vi "Channel 0 Timer And Data Read (SubVI).vi"(5 "BoardHandle in":T1, 7 "Channel # in":i32, 11 "error in (no error)":errorcluster) -> (1 "Actual Voltage Level (V)":dbl format="%#_13g", 2 "Power Supply Trip":bool, 3 "Actual Current Limit (nA)":dbl format="%#_13g", 10 "Array":dbl[](array[numeric]), 14 "BoardHandle out 2":T1, 15 "error out":errorcluster)   [LabVIEW 2020]
uses:
  SUB VI Dark Current Test Files 2018 For Drop Box/Program Files (x86)/National Instruments/LabVIEW 2020/instr.lib/CAEN PSM/CAEN PSM.lvlib
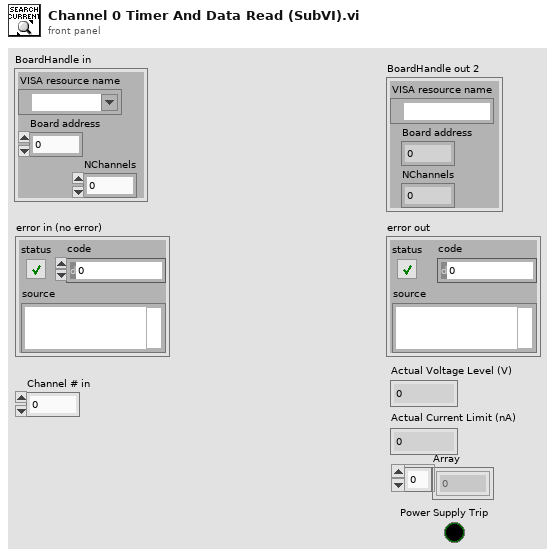
[diagram p1: front panel]
types:
  T1 = cluster{"VISA resource name":refnum<visa-resource-name>, "Board address":u8, "NChannels":u8}
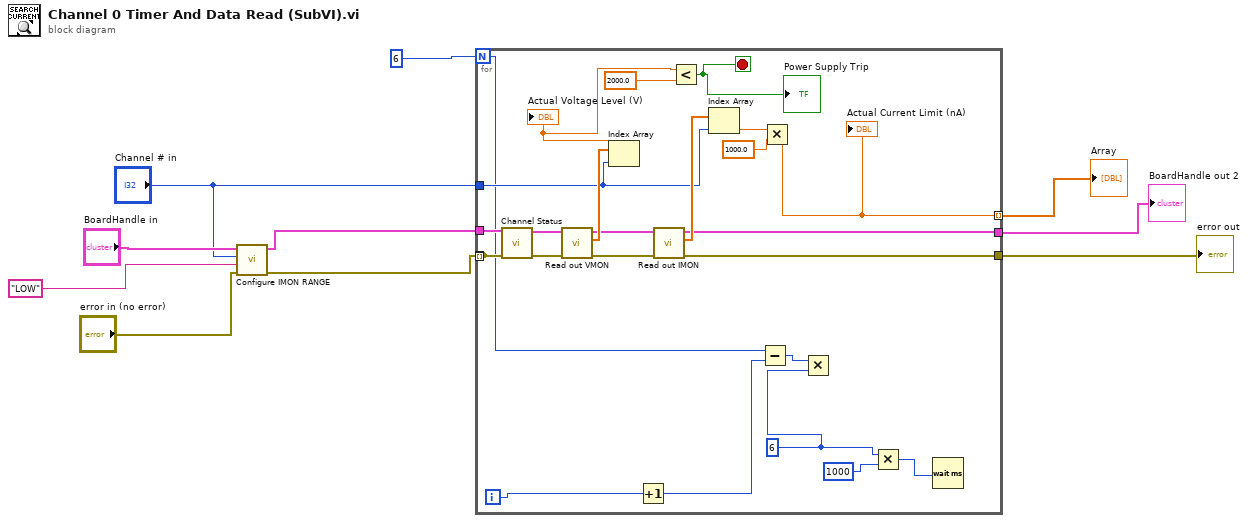
[diagram p0: block diagram]
diagram:
  n1 = call "Configure IMON RANGE.vi"("error in (no error)"="error in (no error)", "IMon range (LOW)"="LOW", "Channel (0)"="Channel # in", "BoardHandle"="BoardHandle in") -> ("error out"=w4:errorcluster, "BoardHandle out"=w5:T1)  [unwired: 6 in]
  n2 = for {
    N: 6 ("N") -> [w18]
    tunnel: w4 -> [w25]
    tunnel: "Channel # in" -> [w26]
    tunnel: [w28] -> w8
    tunnel: [w27] -> w9
    tunnel: [w19] -> w10 mode=indexing
    tunnel: w5 -> [w22]
    tunnel: [w25] -> _ mode=indexing
    i -> [w16]
    stop <- w14 stop-if-true
    w11 = 6 ("dt (s) in")
    n3 = call "Channel Status.vi"("error in (no error)"=w25, "BoardHandle"=w22) -> ("error out"=w34:errorcluster, "BoardHandle out"=w33:T1)  [unwired: 7 in, 1 out]
    n4 = call "Read out VMON.vi"("error in (no error)"=w34, "BoardHandle"=w33) -> ("error out"=w30:errorcluster, "VMon values (V)"=w32:dbl[], "BoardHandle out"=w31:T1)  [unwired: 7 in]
    n5 = Index Array(array=w32, index=w26) -> (element=w13:dbl)
    "Actual Voltage Level (V)" <- w13
    n6 = Increment(x=w16) -> (x+1=w15:i32)
    n7 = call "Read out IMON.vi"("error in (no error)"=w30, "BoardHandle"=w31) -> ("error out"=w27:errorcluster, "IMon values (uA)"=w29:dbl[], "BoardHandle out"=w28:T1)  [unwired: 6 in, 1 out]
    n8 = Less?(x=w13, y=2000.0) -> (x < y?=w14:bool)
    "Power Supply Trip" <- w14
    n9 = Index Array(array=w29, index=w26) -> (element=w21:dbl)
    n10 = Subtract(x=w18, y=w15) -> (x-y=w17:i32)
    n11 = Multiply(x=w21, y=1000.0) -> (x*y=w19:dbl)
    "Actual Current Limit (nA)" <- w19
    n12 = Multiply(x=w17, y=w11) -> ()  [unwired: 1 out]
    n13 = Multiply(x=w11, y=1000) -> (x*y=w24:i32)
    n14 = Wait (ms)(milliseconds to wait=w24) -> ()  [unwired: 1 out]
  }
  "Array" <- w10
  "error out" <- w9
  "BoardHandle out 2" <- w8
